vi "UTILITY Create Nested Directories.vi"(0 "path to create":path, 11 "error in":errorcluster) -> (4 "created path":path, 8 "directory already exists?":bool, 15 "error out":errorcluster)   [LabVIEW 2018]
doc: "This VI creates a set of nested directories specifed by the user. Since the path to the new directories must be absolute (and not relative), the VI will not return an error if some or all of the specified directories already exist. (It also will not alter any pre-existing directories.) \n\nWhen determining the output for DIRECTORY ALREADY EXISTS?, this VI ignores the existence of the root of the path (such as C:\\ )."
panel:
  # "Type the path to create in the string control below. Run."
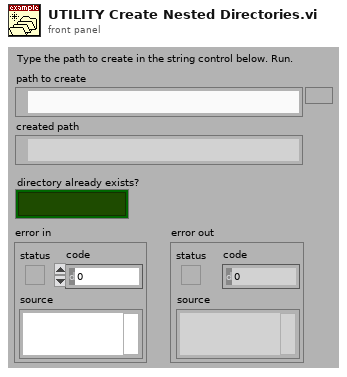
[diagram p1: front panel]
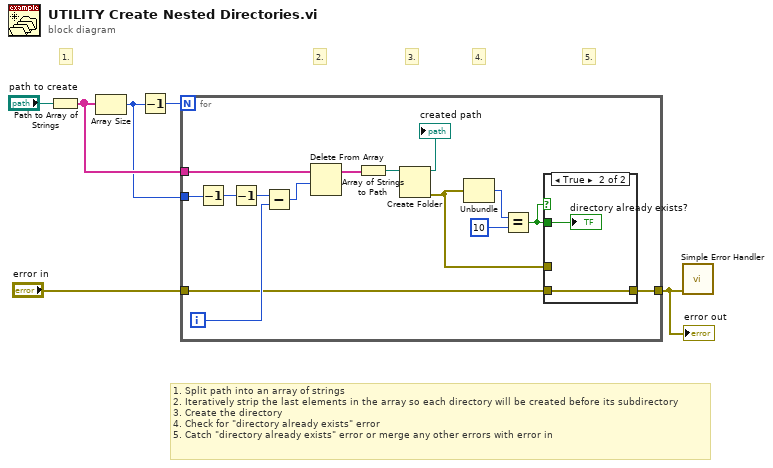
[diagram p0: block diagram]
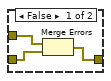
[diagram p2: hidden frame]
diagram:
  # "1. Split path into an array of strings\n2. Iteratively strip the last elements in the array so each directory will be created before its subdirectory\n3. Create the directory\n4. Check for \"directory already exists\" error\n5. Catch \"directory already exists\" error or merge any other errors with error in"
  # "5."
  # "4."
  # "3."
  # "2."
  # "1."
  n1 = Path to Array of Strings(0:"path to create") -> (2:w4:string[])  [unwired: 1 out]
  n2 = Array Size(array=w4) -> (size(s)=w3:i32)
  n3 = Decrement(x=w3) -> (x-1=w5:i32)
  n4 = for {
    N: w5 -> [_]
    tunnel: w4 -> [w21]
    tunnel: w3 -> [w20]
    tunnel: [w10] -> w1
    tunnel: "error in" -> [w9]
    i -> [w15]
    n5 = Decrement(x=w20) -> (x-1=w19:i32)
    n6 = Decrement(x=w19) -> (x-1=w18:i32)
    n7 = Subtract(x=w18, y=w15) -> (x-y=w17:i32)
    n8 = Delete From Array(array=w21, length=w17) -> (array with subset deleted=w16:string[])  [unwired: 1 in, 1 out]
    n9 = Array of Strings to Path(0:w16) -> (2:w8:path)  [unwired: 1 in]
    n10 = Create Folder(path (use dialog)=w8) -> (created path=→"created path":path, error out=w11:errorcluster)  [unwired: 2 in, 1 out]
    n11 = Unbundle(w11) -> ("code"=w14:i32)  [unwired: 2 out]
    n12 = Equal?(x=w14, y=10) -> (x = y?=w12:bool)
    n13 = case shown="True" w12 {
      tunnel: w12 -> [_ w26]
      tunnel: w11 -> [w22 _]
      tunnel: [w24 w25] -> w10
      tunnel: w9 -> [w23 w25]
      frame False {
        n14 = Merge Errors(w22, w23) -> (w24:errorcluster)
      }
      frame True {
        "directory already exists?" <- w26
      }
    }
  }
  "error out" <- w1
  n15 = call <vilib>:"Simple Error Handler.vi"("error in (no error)"=w1) -> ()  [unwired: 4 in, 5 out]
